vi "Estimate total tomo size.vi"(8 "error in (no error)":errorcluster, 11 "Tomo in":refnum<class "Tomo.lvclass">) -> (0 "error out":errorcluster, 2 "filesize in TB":dbl format="%.2f", 3 "Tomo out":refnum<class "Tomo.lvclass">)   [LabVIEW 2012, in "Tomo.lvclass"]
uses:
  Tomo.lvclass
panel:
  out "# frames per tomo":dbl format="%.2f"
  out "frames":dbl format="%.2f"
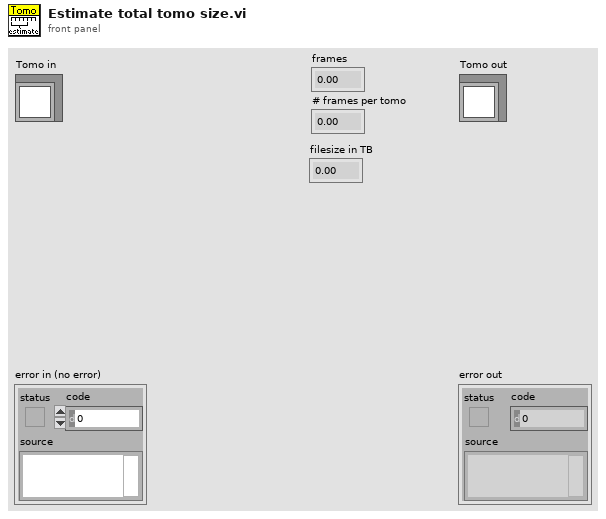
[diagram p1: front panel]
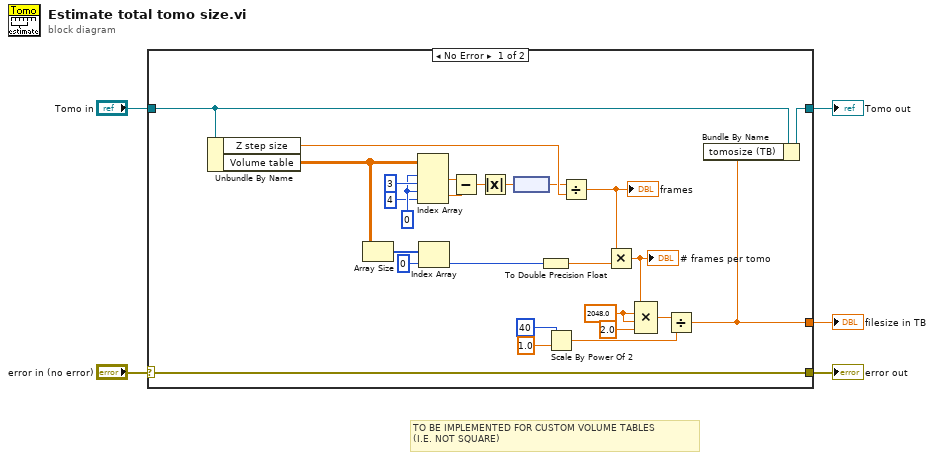
[diagram p0: block diagram]
diagram:
  # "TO BE IMPLEMENTED FOR CUSTOM VOLUME TABLES\n(I.E. NOT SQUARE)"
  n1 = case shown="No Error" "error in (no error)" {
    selector: "error in (no error)" -> [w31 w33]
    tunnel: [w31 w33] -> w4
    tunnel: [w10 w32] -> w2
    tunnel: "Tomo in" -> [w11 w32]
    tunnel: [w9 _] -> w1
    frame No Error {
      w17 = 2048.0
      w29 = 0 ("index (row)")
      n2 = Unbundle By Name(w11) -> ("Z step size"=w24:dbl[unit], "Volume table"=w19:dbl[][])
      n3 = Array Size(array=w19) -> (size(s)=w21:i32[])
      n4 = Index Array(array=w19, index (row) #1=w29, index (col) #1=3 ("disabled index (col)"), index (row) #2=w29, index (col) #2=4 ("disabled index (col)")) -> (element #1=w27:dbl, element #2=w26:dbl)
      n5 = Index Array(array=w21, index=0) -> (element=w18:i32)
      n6 = Subtract(x=w27, y=w26) -> (x-y=w25:dbl)
      n7 = Absolute Value(x=w25) -> (abs(x)=w23:dbl)
      n8 = node(w23) -> (w22:dbl[unit])
      n9 = To Double Precision Float(number=w18) -> (double precision float=w12:dbl)
      n10 = Scale By Power Of 2(n=i16 40, x=1.0) -> (x*2^n=w6:dbl)
      n11 = Divide(x=w22, y=w24) -> (x/y=w13:dbl)
      "frames" <- w13
      n12 = Multiply(x=w13, y=w12) -> (x*y=w15:dbl)
      "# frames per tomo" <- w15
      n13 = Compound Arithmetic op=MULTIPLY(w15, w17, w17, 2.0 ("value")) -> (w14:dbl)
      n14 = Divide(x=w14, y=w6) -> (x/y=w9:dbl)
      n15 = Bundle By Name(cluster=w11, "tomosize (TB)"=w9) -> (w10:refnum<class "Tomo.lvclass">)
    }
    frame Error {
    }
  }
  "error out" <- w4
  "Tomo out" <- w2
  "filesize in TB" <- w1
